vi "read file header.vi"(10 "makeSpeedlinesData in":T1, 11 "Datafiles":path) -> (0 "PR":i32, 1 "massflow":i32, 3 "makeSpeedlinesData out":T1)   [LabVIEW 2018]
uses:
  make speedlines UI data.ctl
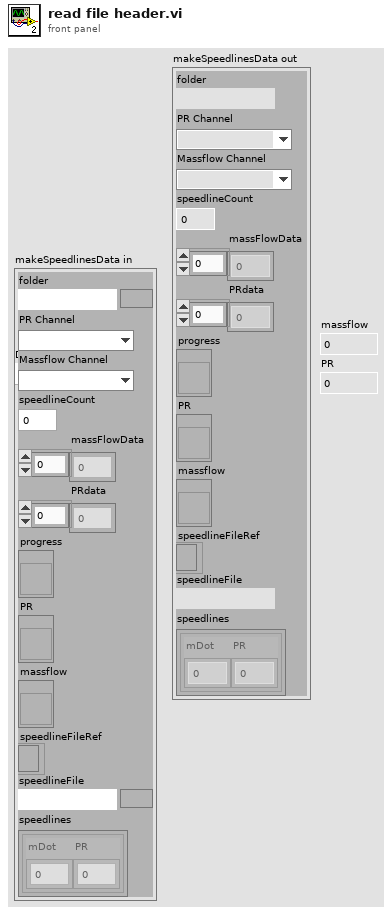
[diagram p1: front panel]
types:
  T1 = typedef "make speedlines UI data.ctl" = cluster{"folder":path, "PR Channel":u16, "Massflow Channel":u16, "speedlineCount":u16, "massFlowData":dbl[], "PRdata":dbl[], "progress":refnum<vi>, "PR":refnum<vi>, "massflow":refnum<vi>, "speedlineFileRef":refnum<file>, "speedlineFile":path, "speedlines":cluster{"mDot":dbl[], "PR":dbl[]}[]}
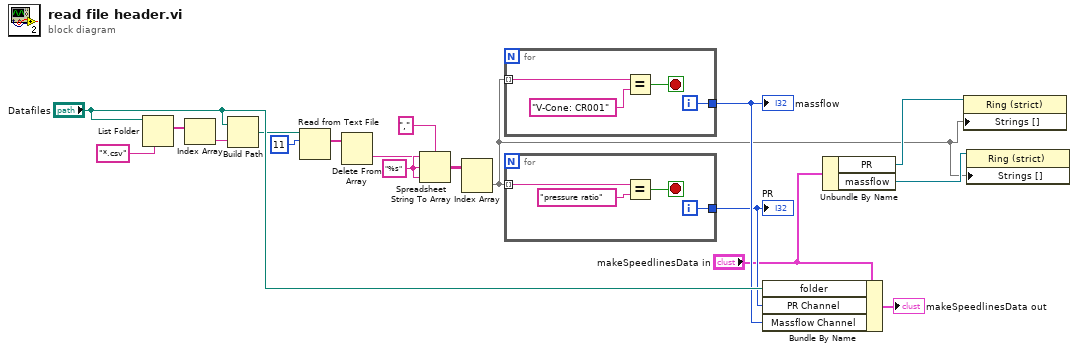
[diagram p0: block diagram]
diagram:
  w2 = "%s" ("spreadsheet string")
  n1 = List Folder(path="Datafiles", pattern="*.csv") -> (filenames=w12:string[])  [unwired: 2 in, 3 out]
  n2 = Index Array(array=w12) -> (element=w13:string)  [unwired: 1 in]
  n3 = Build Path(base path="Datafiles", name or relative path=w13) -> (appended path=w14:path)
  n4 = Read from Text File(file (use dialog)=w14, count=11) -> (text=w16:string[])  [unwired: 2 in, 3 out]
  n5 = Delete From Array(array=w16) -> (deleted portion=w1:string)  [unwired: 2 in, 1 out]
  n6 = Spreadsheet String To Array(delimiter (Tab)=",", format string=w2, spreadsheet string=w1, array type (2D Dbl)=w2) -> (array=w10:string[][])
  n7 = Index Array(array=w10) -> (element=w4:string[])  [unwired: 2 in]
  n8 = for {
    tunnel: w4 -> [w22] mode=indexing
    tunnel: [w20] -> w9
    i -> [w20]
    stop <- w19 stop-if-true
    n9 = Equal?(x=w22, y="V-Cone: CR001" ("spreadsheet string")) -> (x = y?=w19:bool)
  }
  "massflow" <- w9
  n10 = for {
    tunnel: w4 -> [w26] mode=indexing
    tunnel: [w24] -> w8
    i -> [w24]
    stop <- w23 stop-if-true
    n11 = Equal?(x=w26, y="pressure ratio" ("spreadsheet string")) -> (x = y?=w23:bool)
  }
  "PR" <- w8
  n12 = Bundle By Name(cluster="makeSpeedlinesData in", "folder"="Datafiles", "PR Channel"=w8, "Massflow Channel"=w9) -> (→"makeSpeedlinesData out":T1)
  n13 = Unbundle By Name("makeSpeedlinesData in") -> ("PR"=w6:refnum<vi>, "massflow"=w5:refnum<vi>)
  n14 = property class="Ring (strict)"(reference=w6, "Strings []"=w4) -> ()  [unwired: 1 in, 2 out]
  n15 = property class="Ring (strict)"(reference=w5, "Strings []"=w4) -> ()  [unwired: 1 in, 2 out]
